vi "Write Startup Views.vi"(8 "error in (no error)":errorcluster, 9 "View Labels":string[](array[string]), 10 "Startup Views":refnum<class "IViewable.lvclass">[](array[class]), 11 "IViewManager in":refnum<class "IViewManager.lvclass">) -> (0 "error out":errorcluster, 3 "IViewManager out":refnum<class "IViewManager.lvclass">)   [LabVIEW 2015, in "IViewManager.lvlib" / "IViewManager.lvclass"]
doc: "<License>\nCopyright © 2017 Composed Systems, LLC | All rights reserved\nwww.composed.io\n\nAuthor: Ethan Stern <ethan.stern@composed.io>\n\nThis software is provided \"AS IS\" WITHOUT WARRANTIES, either express or implied, AND IS FOR EDUCATIONAL PURPOSES ONLY.\n</License>"
uses:
  IViewManager.lvclass
  IViewable/IViewable/IViewable.lvclass
  IViewManager Messages/Launch Nested Views Msg/Launch Nested Views Msg.lvclass/Launch Nested Views Msg.ctl
  IViewManager.lvclass/IViewManager.ctl
  IViewManager Messages/Launch Nested Views Msg/Launch Nested Views Msg.lvclass
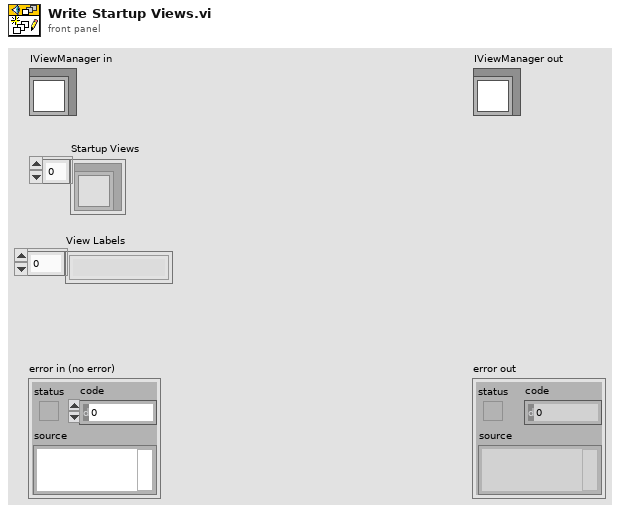
[diagram p1: front panel]
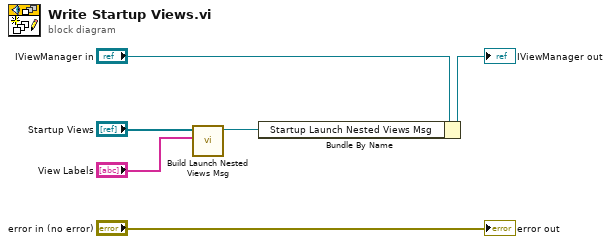
[diagram p0: block diagram]
diagram:
  n1 = call "Build Launch Nested Views Msg.vi"("View Labels"="View Labels", "Nested Views"="Startup Views") -> ("Launch Nested Views Msg out"=w1:refnum<class "Launch Nested Views Msg.lvclass">)  [unwired: 8 in, 1 out]
  n2 = Bundle By Name(cluster="IViewManager in", "Startup Launch Nested Views Msg"=w1) -> (→"IViewManager out":refnum<class "IViewManager.lvclass">)
  "error out" <- "error in (no error)"
